vi "getPath.vi"(0 "reference":refnum<class "BentStyle.lvclass">, 1 "start":T2 {"height" format="%.2f"; "width" format="%.2f"; "y" format="%.2f"; "x" format="%.2f"}, 2 "end":T2 {"height" format="%.2f"; "width" format="%.2f"; "y" format="%.2f"; "x" format="%.2f"}, 5 "error in (no error)":errorcluster) -> (14 "reference out":refnum<class "BentStyle.lvclass">, 15 "path":T3[](array[typedef]) {"y" format="%.2f"; "x" format="%.2f"}, 16 "startDirection":T1, 17 "endDirection":T1, 19 "error out":errorcluster)   [LabVIEW 2020, in "BentStyle.lvclass"]
doc: "/**\n Gets the points at which a line joining two rectangles\n is bent according to this bent style.\n @param start the starting rectangle\n @param end the ending rectangle\n @return an array list of points at which to bend the\n segmented line joining the two rectangles\n */\n public ArrayList getPath(Rectangle2D start, Rectangle2D end)"
uses:
  <resource>/Framework/Providers/Open_GDS/UML/BentStyle_class/BentStyle.lvclass
  <resource>/Framework/Providers/Open_GDS/UML/General/Point/Point Point2D.ctl
  <resource>/Framework/Providers/Open_GDS/UML/General/Rectangle/Rectangle Rectangle2D.ctl
  <resource>/Framework/Providers/Open_GDS/UML/Direction_class/DirectionTypes.ctl
  <resource>/Framework/Providers/Open_GDS/UML/BentStyle_class/BentStyle.lvclass/BentStyle.ctl
  <resource>/Framework/Providers/Open_GDS/UML/BentStyle_class/BentStyleType.ctl
  <resource>/Framework/Providers/Open_GDS/UML/Direction_class/Direction.lvclass
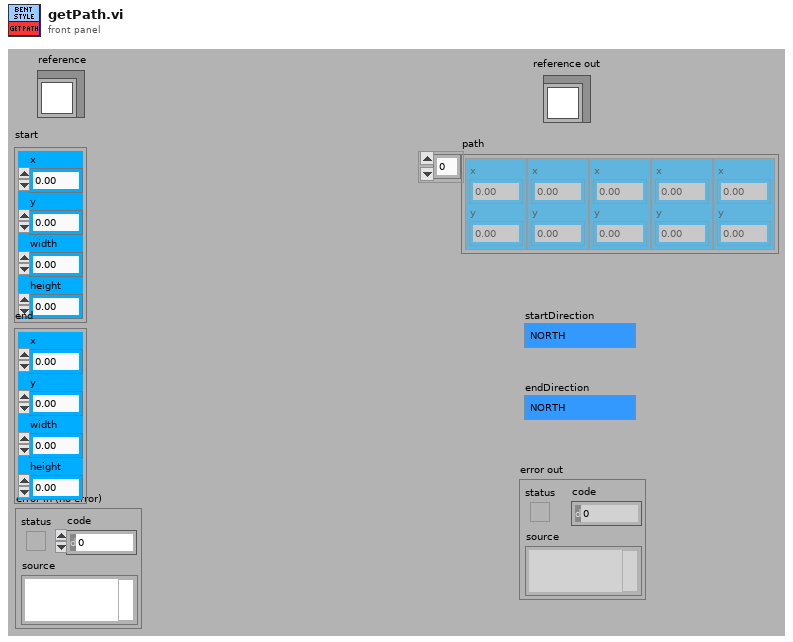
[diagram p1: front panel]
types:
  T1 = typedef "Direction.lvclass/DirectionTypes.ctl" = enum16{"NORTH", "SOUTH", "EAST", "WEST"}
  T2 = typedef "Rectangle Rectangle2D.ctl" = cluster{"x":dbl, "y":dbl, "width":dbl, "height":dbl}
  T3 = typedef "Point Point2D.ctl" = cluster{"x":dbl, "y":dbl}
  T4 = typedef "BentStyle.lvclass/BentStyleType.ctl" = enum16{"STRAIGHT", "HV", "VH", "HVH", "VHV", "ARC"}
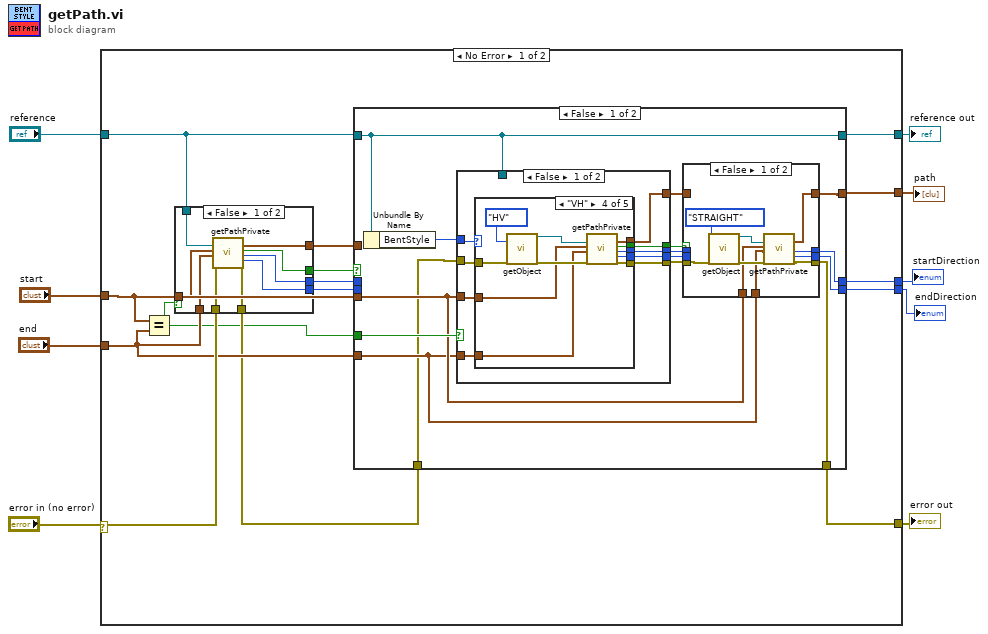
[diagram p0: block diagram]
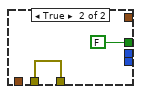
[diagram p2: hidden frame]
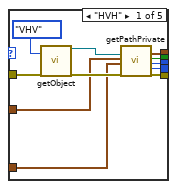
[diagram p4: hidden frame]
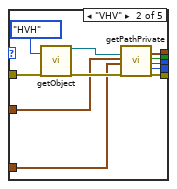
[diagram p5: hidden frame]
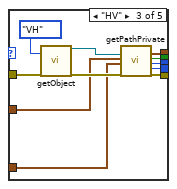
[diagram p6: hidden frame]
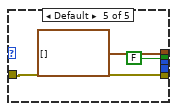
[diagram p7: hidden frame]
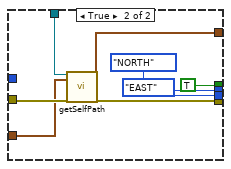
[diagram p8: hidden frame]
diagram:
  n1 = case shown="No Error" "error in (no error)" {
    selector: "error in (no error)" -> [w22 w134]
    tunnel: "reference" -> [w10 w135]
    tunnel: [w24 w134] -> w8
    tunnel: [w23 w135] -> w7
    tunnel: "start" -> [w21 _]
    tunnel: "end" -> [w20 _]
    tunnel: [w19 _] -> w3
    tunnel: [w18 _] -> w2
    tunnel: [w17 _] -> w1
    frame No Error {
      n2 = Equal?(x=w21, y=w20) -> (x = y?=w11:bool)
      n3 = case shown="False" w11 {
        tunnel: w22 -> [w33 w35]
        tunnel: [w32 _] -> w16
        tunnel: w10 -> [w31 _]
        tunnel: [w30 w35] -> w15
        tunnel: w21 -> [w29 _]
        tunnel: w20 -> [w28 _]
        tunnel: [w27 FALSE ("ok")] -> w14
        tunnel: [w26 _] -> w13
        tunnel: [w25 _] -> w12
        frame False {
          n4 = call <resource>:"getPathPrivate.vi"("bentStyleRef"=w31, "start"=w29, "end"=w28, "error in (no error)"=w33) -> ("path"=w32:T3[], "ok"=w27:bool, "startDirection"=w26:T1, "endDirection"=w25:T1, "error out"=w30:errorcluster)  [unwired: 11 out]
        }
        frame True {
        }
      }
      n5 = case shown="False" w14 {
        tunnel: w16 -> [_ w133]
        tunnel: [w45 w133] -> w19
        tunnel: w10 -> [w36 w129]
        tunnel: [w36 w129] -> w23
        tunnel: w15 -> [w37 w132]
        tunnel: w11 -> [w50 _]
        tunnel: [w46 w132] -> w24
        tunnel: w21 -> [w44 _]
        tunnel: w20 -> [w43 _]
        tunnel: [w42 w131] -> w18
        tunnel: w13 -> [_ w131]
        tunnel: [w41 w130] -> w17
        tunnel: w12 -> [_ w130]
        frame False {
          n6 = Unbundle By Name(w36) -> ("BentStyle"=w38:T4)
          n7 = case shown="False" w50 {
            tunnel: w37 -> [w72 w128]
            tunnel: [w71 w127] -> w47
            tunnel: [w68 w126] -> w48
            tunnel: w44 -> [w70 w125]
            tunnel: w38 -> [w73 _]
            tunnel: w43 -> [w69 _]
            tunnel: w36 -> [_ w124]
            tunnel: [w67 TRUE ("ok")] -> w49
            tunnel: [w66 DirectionTypes."NORTH" ("startDirection")] -> w40
            tunnel: [w65 DirectionTypes."EAST" ("startDirection")] -> w39
            frame False {
              n8 = case shown="\"VH\"" w73 {
                tunnel: w72 -> [w83 w94 w105 w116 w118]
                tunnel: [w82 w93 w104 w115 w118] -> w71
                tunnel: w70 -> [w79 w90 w101 w112 _]
                tunnel: w69 -> [w78 w89 w100 w111 _]
                tunnel: [w77 w88 w99 w110 T3[] [] ("path")] -> w68
                tunnel: [w76 w87 w98 w109 FALSE ("ok")] -> w67
                tunnel: [w75 w86 w97 w108 _] -> w66
                tunnel: [w74 w85 w96 w107 _] -> w65
                frame "HVH" {
                  n9 = call <resource>:"getObject.vi"("bentStyle"=BentStyleType."VHV", "error in (no error)"=w83) -> ("reference out"=w80:refnum<class "BentStyle.lvclass">, "error out"=w84:errorcluster)  [unwired: 16 out]
                  n10 = call <resource>:"getPathPrivate.vi"("bentStyleRef"=w80, "start"=w79, "end"=w78, "error in (no error)"=w84) -> ("path"=w77:T3[], "ok"=w76:bool, "startDirection"=w75:T1, "endDirection"=w74:T1, "error out"=w82:errorcluster)  [unwired: 11 out]
                }
                frame "VHV" {
                  n11 = call <resource>:"getObject.vi"("bentStyle"=BentStyleType."HVH", "error in (no error)"=w94) -> ("reference out"=w91:refnum<class "BentStyle.lvclass">, "error out"=w95:errorcluster)  [unwired: 16 out]
                  n12 = call <resource>:"getPathPrivate.vi"("bentStyleRef"=w91, "start"=w90, "end"=w89, "error in (no error)"=w95) -> ("path"=w88:T3[], "ok"=w87:bool, "startDirection"=w86:T1, "endDirection"=w85:T1, "error out"=w93:errorcluster)  [unwired: 11 out]
                }
                frame "HV" {
                  n13 = call <resource>:"getObject.vi"("bentStyle"=BentStyleType."VH", "error in (no error)"=w105) -> ("reference out"=w102:refnum<class "BentStyle.lvclass">, "error out"=w106:errorcluster)  [unwired: 16 out]
                  n14 = call <resource>:"getPathPrivate.vi"("bentStyleRef"=w102, "start"=w101, "end"=w100, "error in (no error)"=w106) -> ("path"=w99:T3[], "ok"=w98:bool, "startDirection"=w97:T1, "endDirection"=w96:T1, "error out"=w104:errorcluster)  [unwired: 11 out]
                }
                frame "VH" {
                  n15 = call <resource>:"getObject.vi"("bentStyle"=BentStyleType."HV", "error in (no error)"=w116) -> ("reference out"=w113:refnum<class "BentStyle.lvclass">, "error out"=w117:errorcluster)  [unwired: 16 out]
                  n16 = call <resource>:"getPathPrivate.vi"("bentStyleRef"=w113, "start"=w112, "end"=w111, "error in (no error)"=w117) -> ("path"=w110:T3[], "ok"=w109:bool, "startDirection"=w108:T1, "endDirection"=w107:T1, "error out"=w115:errorcluster)  [unwired: 11 out]
                }
                frame Default {
                }
              }
            }
            frame True {
              n17 = call <resource>:"getSelfPath.vi"("reference"=w124, "bounds"=w125, "error in (no error)"=w128) -> ("path"=w126:T3[], "error out"=w127:errorcluster)  [unwired: 15 out]
            }
          }
          n18 = case shown="False" w49 {
            tunnel: w48 -> [_ w63]
            tunnel: w47 -> [w58 w64]
            tunnel: [w55 w64] -> w46
            tunnel: [w56 w63] -> w45
            tunnel: w44 -> [w54 _]
            tunnel: w43 -> [w53 _]
            tunnel: [w52 w62] -> w42
            tunnel: [w51 w61] -> w41
            tunnel: w40 -> [_ w62]
            tunnel: w39 -> [_ w61]
            frame False {
              n19 = call <resource>:"getObject.vi"("bentStyle"=BentStyleType."STRAIGHT", "error in (no error)"=w58) -> ("reference out"=w60:refnum<class "BentStyle.lvclass">, "error out"=w59:errorcluster)  [unwired: 16 out]
              n20 = call <resource>:"getPathPrivate.vi"("bentStyleRef"=w60, "start"=w54, "end"=w53, "error in (no error)"=w59) -> ("path"=w56:T3[], "startDirection"=w52:T1, "endDirection"=w51:T1, "error out"=w55:errorcluster)  [unwired: 12 out]
            }
            frame True {
            }
          }
        }
        frame True {
        }
      }
    }
    frame Error {
    }
  }
  "reference out" <- w7
  "error out" <- w8
  "path" <- w3
  "startDirection" <- w2
  "endDirection" <- w1
